vi "C.vi"(8 "error in (no error)":errorcluster) -> (0 "C error out":errorcluster)   [LabVIEW 2017]
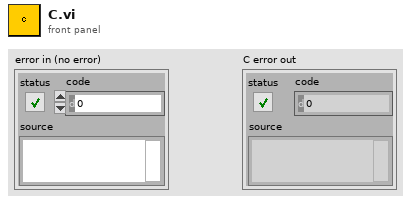
[diagram p1: front panel]
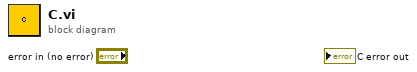
[diagram p0: block diagram]
diagram:
